vi "Get Voltage RGB.vi"(3 "error in (no error)":errorcluster, 4 "Voltage":dbl, 5 "ColorRamp in":refnum<vi>) -> (0 "error out":errorcluster, 1 "RGB Value":u32, 2 "ColorRamp out":refnum<vi>)   [LabVIEW 2020]
doc: "This VI gets a color value (RGB) from a voltage."
panel:
  out "Color Box":u32(colorbox)
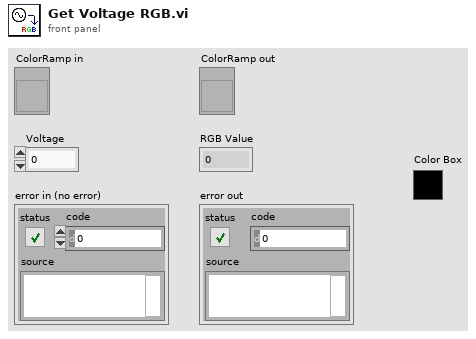
[diagram p1: front panel]
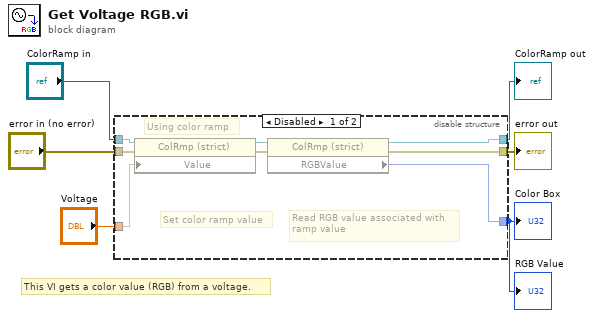
[diagram p0: block diagram]
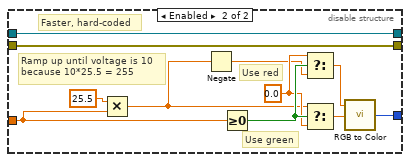
[diagram p2: hidden frame]
diagram:
  # "This VI gets a color value (RGB) from a voltage."
  n1 = disable-structure shown="Disabled" {
    disable-tunnel: [w14 w25] -> w1
    disable-tunnel: "Voltage" -> [w12 w21]
    disable-tunnel: "error in (no error)" -> [w10 w23]
    disable-tunnel: "ColorRamp in" -> [w9 w24]
    disable-tunnel: [w8 w24] -> w3
    disable-tunnel: [w7 w23] -> w2
    frame Disabled {
      # "Read RGB value associated with\nramp value"
      # "Set color ramp value"
      # "Using color ramp"
      n2 = property class="ColRmp (strict)"(reference=w9, error in=w10, "Value"=w12) -> (reference out=w11:refnum<vi>, error out=w13:errorcluster)
      n3 = property class="ColRmp (strict)"(reference=w11, error in=w13) -> (reference out=w8:refnum<vi>, error out=w7:errorcluster, "RGBValue"=w14:u32)
    }
    frame Enabled {
      w17 = 0.0 ("f")
      # "Use red"
      # "Use green"
      # "Ramp up until voltage is 10\nbecause 10*25.5 = 255"
      # "Faster, hard-coded"
      n4 = Multiply(x=25.5, y=w21) -> (x*y=w16:dbl)
      n5 = Negate(x=w16) -> (-x=w15:dbl)
      n6 = Greater Or Equal To 0?(x=w21) -> (x >= 0?=w19:bool)
      n7 = Select(t=w17, s=w19, f=w15) -> (s? t:f=w18:dbl)
      n8 = Select(t=w16, s=w19, f=w17) -> (s? t:f=w20:dbl)
      n9 = call <vilib>:"RGB to Color.vi"("G"=w20, "R"=w18) -> ("Color"=w25:u32)  [unwired: 1 in]
    }
  }
  "RGB Value" <- w1
  "ColorRamp out" <- w3
  "error out" <- w2
  "Color Box" <- w1
